vi "Introduccion_a_labView.vi"() -> ()   [LabVIEW 2019]
panel:
  in  "Slide 2":dbl(slide) scale=0.0..10.0
  out "Slide 3":dbl(slide) scale=0.0..20.0
  in  "Slide":dbl(slide) scale=0.0..10.0
  out "Gauge":dbl(knob) scale=0.0..10.0
  in  "Knob":dbl(knob) scale=0.0..10.0
  out "Boolean 2":bool
  in  "Boolean":bool
  in  "Interruptor 3":bool
  out "LED 3":bool
  in  "Interruptor 2":bool
  out "LED 2":bool
  in  "Interruptor 1":bool
  out "LED":bool
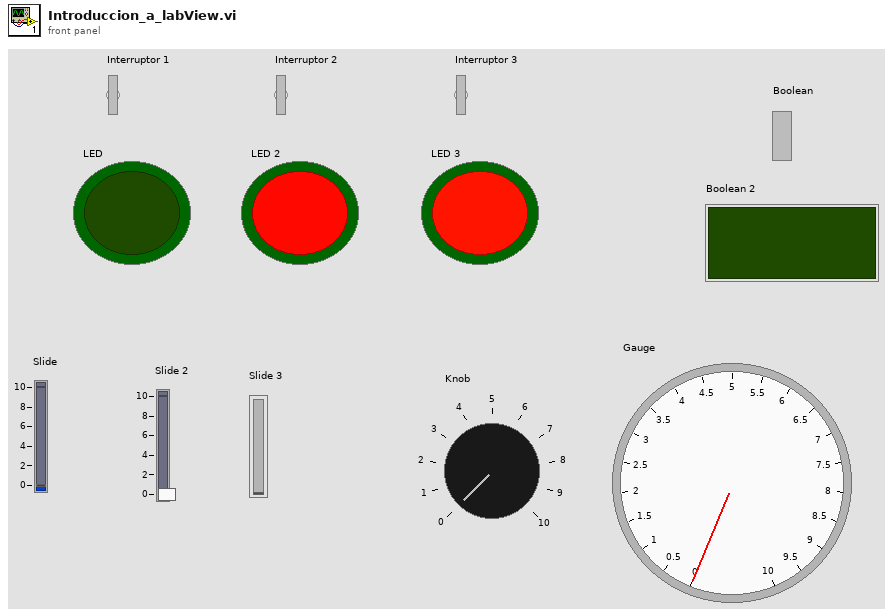
[diagram p1: front panel]
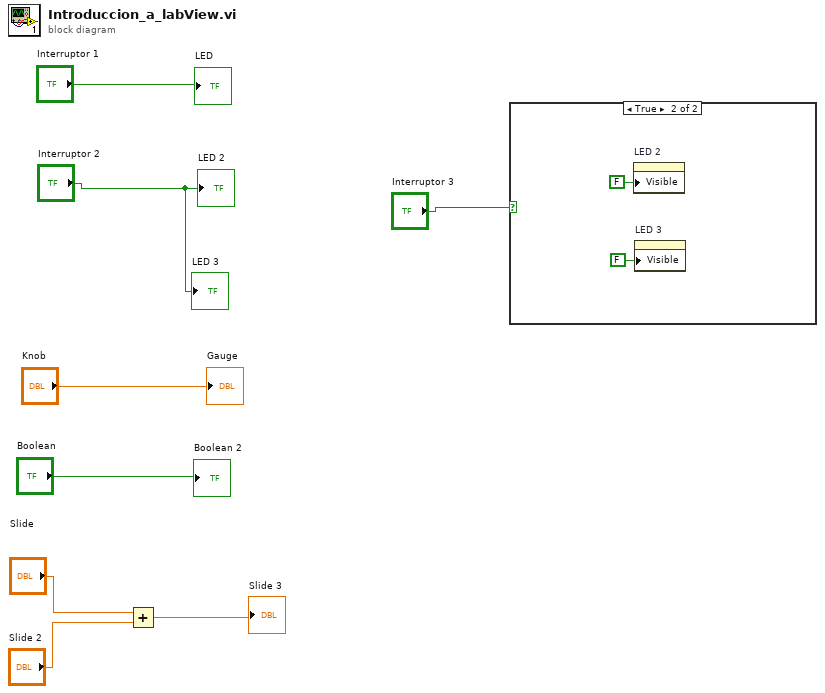
[diagram p0: block diagram]
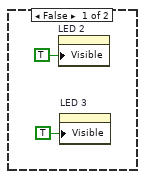
[diagram p2: hidden frame]
diagram:
  n1 = Add(x="Slide", y="Slide 2") -> (x+y=→"Slide 3":dbl)
  n2 = case shown="True" "Interruptor 3" {
    frame False {
      n3 = property on="LED 2" class="Bool (strict)"("Visible"=TRUE) -> ()  [unwired: 2 in, 2 out]
      n4 = property on="LED 3" class="Bool (strict)"("Visible"=TRUE) -> ()  [unwired: 2 in, 2 out]
    }
    frame True {
      n5 = property on="LED 2" class="Bool (strict)"("Visible"=FALSE) -> ()  [unwired: 2 in, 2 out]
      n6 = property on="LED 3" class="Bool (strict)"("Visible"=FALSE) -> ()  [unwired: 2 in, 2 out]
    }
  }
  "LED" <- "Interruptor 1"
  "LED 2" <- "Interruptor 2"
  "LED 3" <- "Interruptor 2"
  "Boolean 2" <- "Boolean"
  "Gauge" <- "Knob"
